vi "PRL UTIL Check Time Stamp Age.vi"(10 "Max Age Allowed [s]":dbl=1.0, 11 "Time Stamp to Check":timestamp) -> (2 "Trigger":bool, 3 "Latest Time Stamp":timestamp)   [LabVIEW 2013, in "PMU Recorder Light.lvlib"]
uses:
  PMU Recorder Light.lvlib
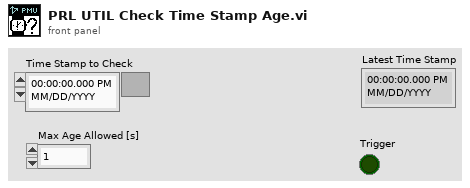
[diagram p1: front panel]
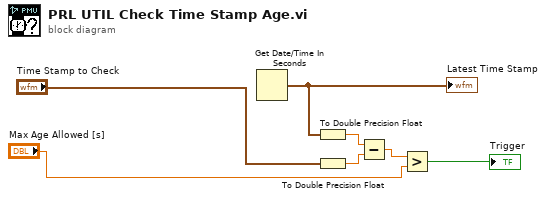
[diagram p0: block diagram]
diagram:
  n1 = Get Date/Time In Seconds() -> (seconds since 1Jan1904=w1:timestamp)
  "Latest Time Stamp" <- w1
  n2 = To Double Precision Float(number=w1) -> (double precision float=w5:dbl)
  n3 = To Double Precision Float(number="Time Stamp to Check") -> (double precision float=w6:dbl)
  n4 = Subtract(x=w5, y=w6) -> (x-y=w7:dbl)
  n5 = Greater?(x=w7, y="Max Age Allowed [s]") -> (0:→"Trigger":bool)
